vi "DATOS ESCRITOS.vi"() -> ()   [LabVIEW 2020]
panel:
  out "GRAFICO DE LA SEÑAL":dynamicdata(graph)
  in  "STOP":bool
  out "ALARMA":bool
  in  "LIM":dbl
  in  "TEMP":dbl
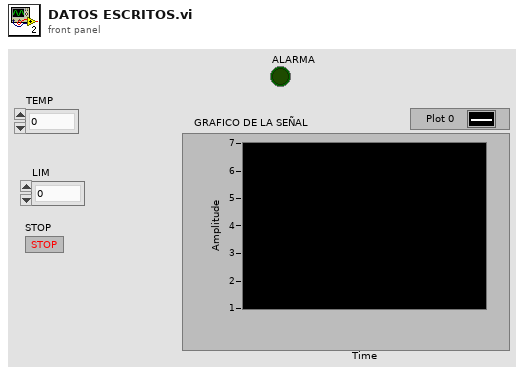
[diagram p1: front panel]
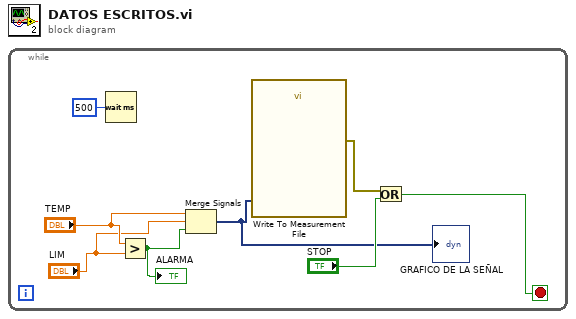
[diagram p0: block diagram]
diagram:
  n1 = while {
    stop <- w2 stop-if-true
    n2 = Wait (ms)(milliseconds to wait=u32 500) -> ()  [unwired: 1 out]
    n3 = Greater?(x="TEMP", y="LIM") -> (0:w5:bool)
    "ALARMA" <- w5
    n4 = Merge Signals("TEMP", "LIM", w5) -> (w1:dynamicdata)
    "GRAFICO DE LA SEÑAL" <- w1
    n5 = call "Write To Measurement File"("Signals"=w1) -> ("error out"=w4:errorcluster)  [unwired: 16 in, 2 out]
    n6 = Or(x=w4, y="STOP") -> (x .or. y?=w2:bool)
  }
